vi "FT10_Serial Number.vi"() -> (2 "Generator Serial Number out":T1)   [LabVIEW 2015]
uses:
  Controls/Control_Serial Number.ctl
panel:
  in  "Generator Serial Number in":T1
  in  "OK Button":bool
  # "Enter Serial Number"
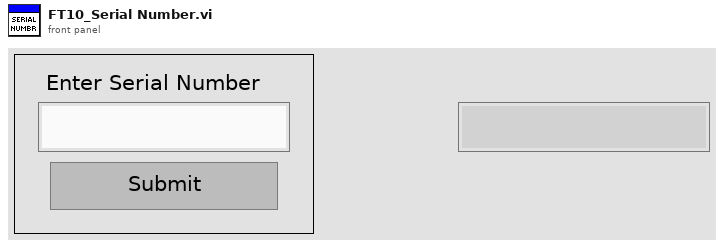
[diagram p1: front panel]
types:
  T1 = typedef "Control_Serial Number.ctl" = string
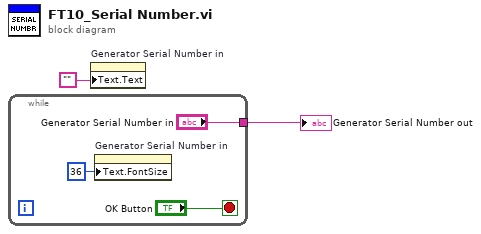
[diagram p0: block diagram]
diagram:
  n1 = while {
    tunnel: ["Generator Serial Number in"] -> w1
    stop <- "OK Button" stop-if-true
    n2 = property on="Generator Serial Number in" class="Str (strict)"("Text.FontSize"=u32 36 ("Text.Font:Size")) -> ()  [unwired: 2 in, 2 out]
  }
  "Generator Serial Number out" <- w1
  n3 = property on="Generator Serial Number in" class="Str (strict)"("Text.Text"="") -> ()  [unwired: 2 in, 2 out]
